vi "Converting data from file to table.vi"() -> ()   [LabVIEW 2024]
panel:
  out "array":string[][](array[string])
  out "text":string
  in  "Path":path
  out "Table Control":string[][](table)
  # "Overview:\n1. In this VI,  all the values in a text file were converted to table format in the front panel.\nI will explain all the functions and controls used in this.\n1. Table Control is  in the Control ->controls->list,table,Tree(refer to the image on sliding front panel to the left.)\nBlock diagram:\n1. Path: to add teh path that the text file is stored. functions->string>path\n2. Build path is the File I/O.\n3. Open file read file and close file  all are from file I/O.\n4. string text to read teh text fromthe read file palette.\n5. Spreadsheet to string array and array subset are from the arrays palette.\n6. Index array is chosed to add the headers to the table.\n7.  property node used in this column Header strings to add header to the table,"
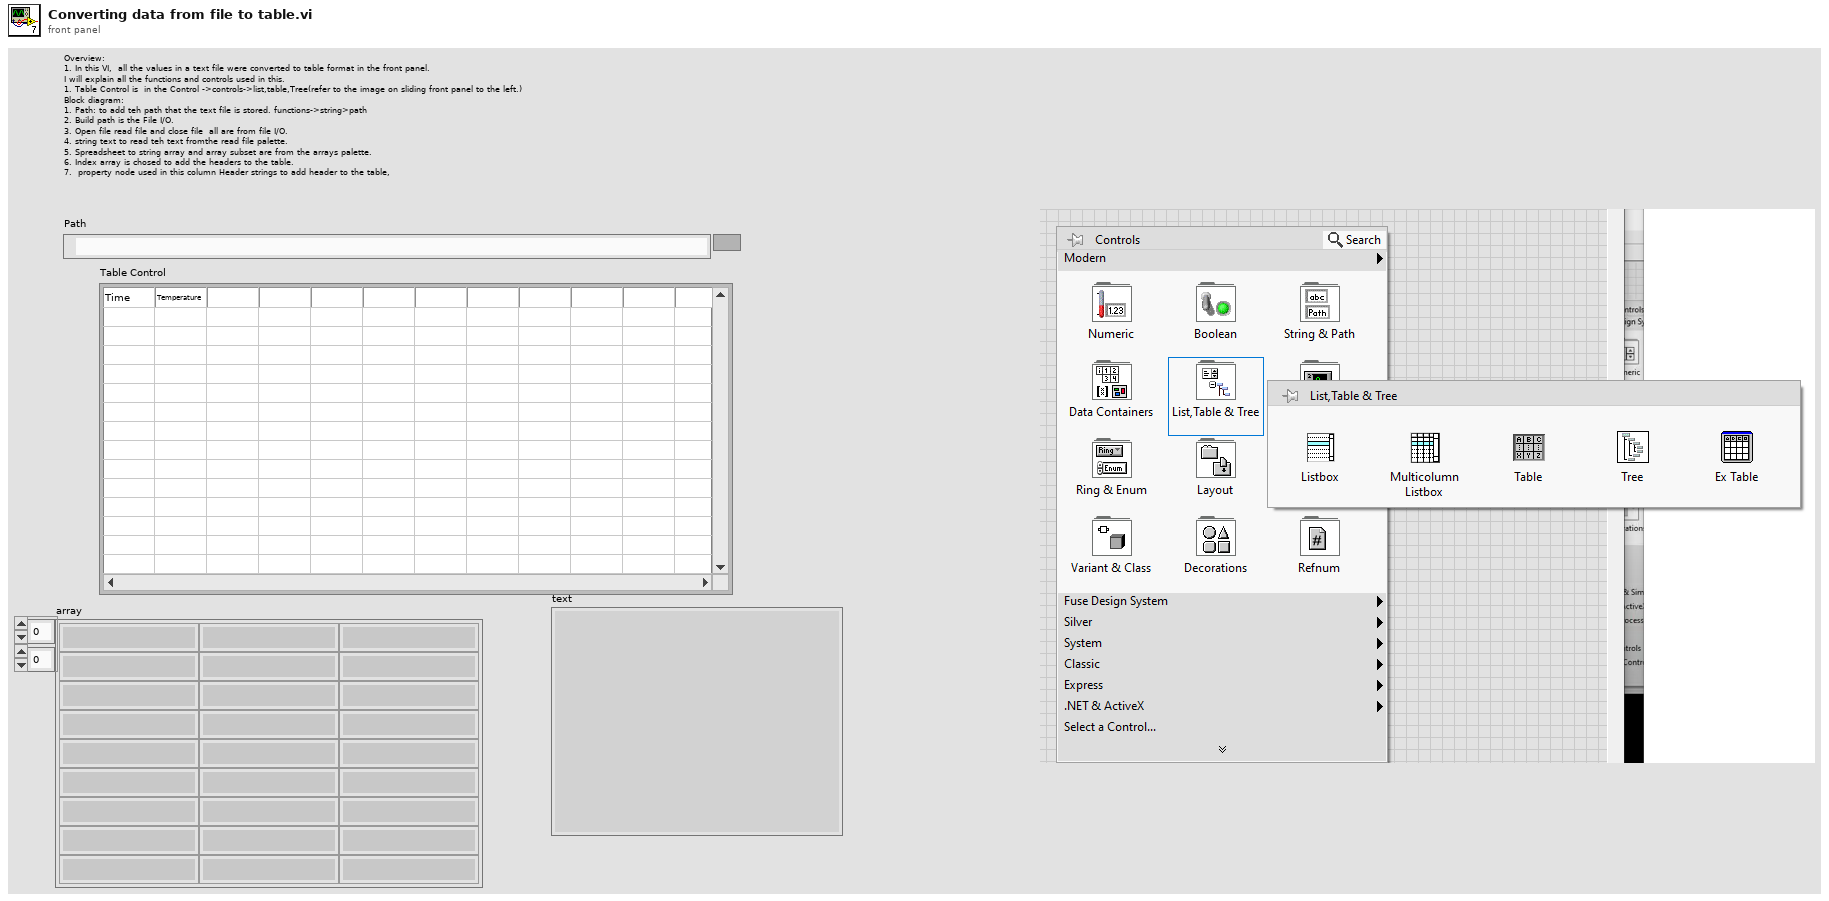
[diagram p1: front panel]
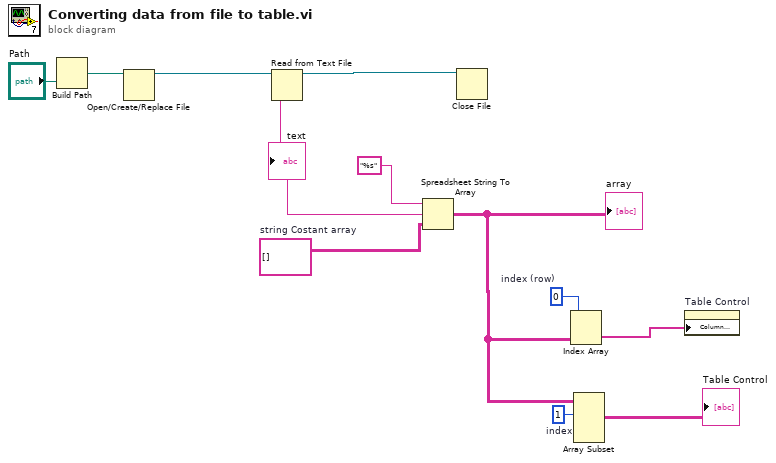
[diagram p0: block diagram]
diagram:
  w2 = 1  # index
  w5 = 0  # index (row)
  w7 = string[][] []  # string Costant array
  n1 = Build Path(name or relative path="Path") -> (appended path=w11:path)  [unwired: 1 in]
  n2 = Open/Create/Replace File(file path (use dialog)=w11) -> (refnum out=w10:refnum<file>)  [unwired: 5 in, 2 out]
  n3 = Read from Text File(file (use dialog)=w10) -> (refnum out=w9:refnum<file>, text=w6:string)  [unwired: 3 in, 2 out]
  "text" <- w6
  n4 = Spreadsheet String To Array(format string="%s" ("delimiter (Tab)"), spreadsheet string=w6, array type (2D Dbl)=w7) -> (array=w3:string[][])  [unwired: 1 in]
  "array" <- w3
  n5 = Close File(refnum=w9) -> ()  [unwired: 1 in, 2 out]
  n6 = Index Array "Index Array"(array=w3, index (row)=w5) -> (element=w4:string[])  [unwired: 1 in]
  n7 = Array Subset "Array Subset"(array=w3, index (row)=w2) -> (→"Table Control":string[][])  [unwired: 3 in]
  n8 = property on="Table Control" class="Tbl (strict)"("Column Headers[]"=w4) -> ()  [unwired: 2 in, 2 out]
